vi "GetNetworkAdapterSettings.vi"(8 "error in (no error)":errorcluster) -> (0 "error out":errorcluster, 3 "Network Adapter Settings":T1[](array[typedef]) {"IP Address Request Mode" items=["Static"=1, "DHCP/Link Local"=2, "Link-Local Only"=4, "DHCP Only"=8]; "Adapter Mode" items=["Disabled"=1, "TCP/IP Ethernet"=2, "Deterministic"=4, "EtherCAT"=8, "TCP/IP WLAN Connect"=32, "TCP/IP WLAN Create"=64]}, 5 "Found?":bool)   [LabVIEW 2017, in "SystemInfoProcess.lvlib"]
doc: "Gets network adapter settings, such as IP address, Gateway, DNS server, and alias."
uses:
  <vilib>/addons/SystemInfoProcess/SystemInfoProcess.lvlib
  <vilib>/addons/SystemInfoProcess/controls/NetworkAdapterSettings.ctl
  <vilib>/addons/PointValueMap/subVIs/Point_Read_variant.vi
  <vilib>/addons/PointValueMap/PointValueMap.lvlib
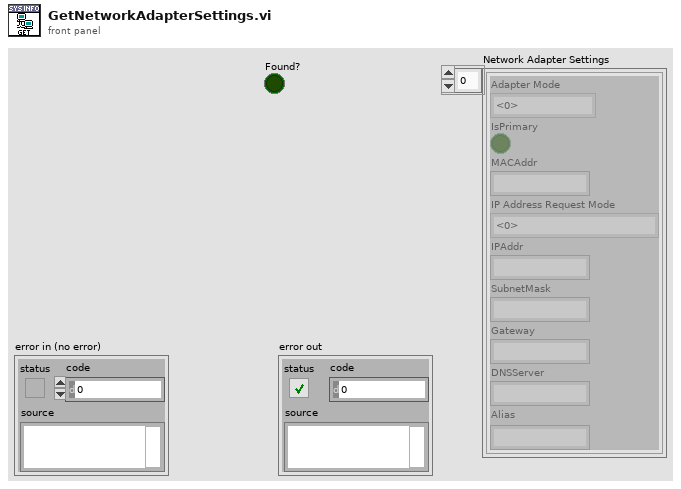
[diagram p1: front panel]
types:
  T1 = typedef "SystemInfoProcess.lvlib/NetworkAdapterSettings.ctl" = cluster{"Adapter Mode":u32, "IsPrimary":bool, "MACAddr":string, "IP Address Request Mode":u32, "IPAddr":string, "SubnetMask":string, "Gateway":string, "DNSServer":string, "Alias":string}
  T2 = typedef "PointValueMap.lvlib/PointMap.ctl" = refnum<data-value>
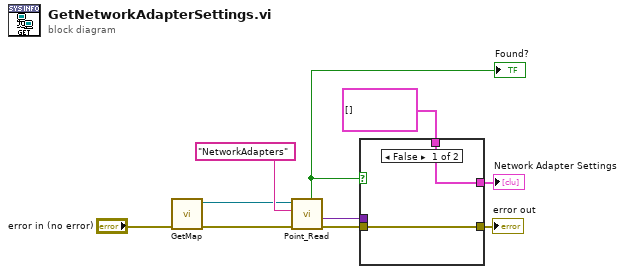
[diagram p0: block diagram]
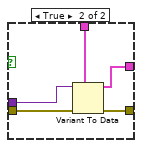
[diagram p2: hidden frame]
diagram:
  n1 = call <vilib>:"GetMap.vi"("error in (no error)"="error in (no error)") -> ("error out"=w3:errorcluster, "SystemInfoMap"=w2:T2)  [unwired: 9 in]
  n2 = call-poly <vilib>:"Point_Read.vi"("Error In"=w3, "Tag"="NetworkAdapters", "Map"=w2) -> ("Error Out"=w10:errorcluster, "Value"=w5:variant, "Valid?"=w4:bool)  [unwired: 3 in, 3 out]
  "Found?" <- w4
  n3 = case shown="False" w4 {
    tunnel: w10 -> [w11 w17]
    tunnel: [w11 w16] -> w9
    tunnel: T1[] [] ("Network Adapter Settings") -> [w12 w15]
    tunnel: [w12 w14] -> w6
    tunnel: w5 -> [_ w13]
    frame False {
    }
    frame True {
      n4 = Variant To Data(error in=w17, type=w15, Variant=w13) -> (data=w14:T1[], error out=w16:errorcluster)
    }
  }
  "error out" <- w9
  "Network Adapter Settings" <- w6
